vi "get#SamplesPerChannel.vi"(8 "error in (no error)":errorcluster, 10 "NIDAQmx data format":digitalwaveform[](array[waveform]), 11 "niDAQmxDO in":refnum<class "niDAQmxDO.lvclass">) -> (0 "error out":errorcluster, 1 "samplesPerChannel":i32, 2 "NIDAQmx data format out":digitalwaveform[](array[waveform]), 3 "niDAQmxDO out":refnum<class "niDAQmxDO.lvclass">)   [LabVIEW 2009, in "Hardware.lvlib" / "Channels.lvlib" / "niDAQmxDO.lvclass"]
uses:
  niDAQmxDO.lvclass
  <vilib>/Waveform/DWDTOps.llb/DWDT Digital to Boolean Array.vi
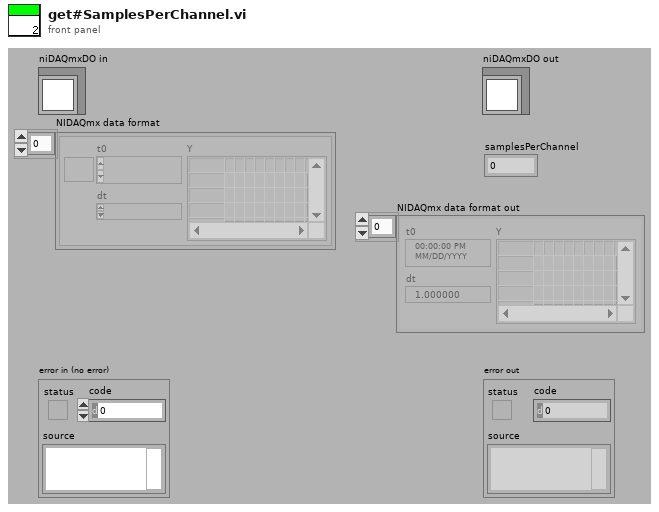
[diagram p1: front panel]
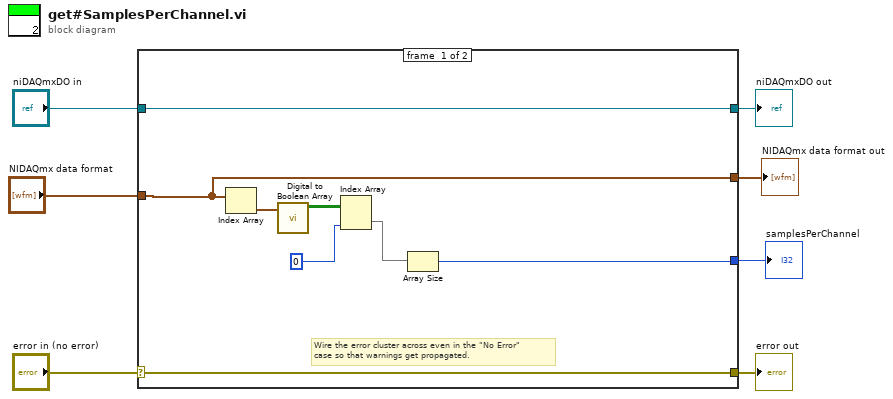
[diagram p0: block diagram]
diagram:
  n1 = case shown="No Error" "error in (no error)" {
    selector: "error in (no error)" -> [w14 w17]
    tunnel: [w14 w17] -> w6
    tunnel: [w15 w16] -> w4
    tunnel: "niDAQmxDO in" -> [w15 w16]
    tunnel: "NIDAQmx data format" -> [w8 _]
    tunnel: [w9 _] -> w2
    tunnel: [w8 _] -> w1
    frame #0 {
      # "Wire the error cluster across even in the \"No Error\"\ncase so that warnings get propagated."
      n2 = Index Array(array=w8) -> (element=w13:digitalwaveform)  [unwired: 1 in]
      n3 = call-poly <vilib>:"Digital to Boolean Array.vi"("digital waveform"=w13) -> ("boolean array"=w12:bool[][])  [unwired: 9 in, 1 out]
      n4 = Index Array(array=w12, index (col)=0) -> (element=w10:bool[])  [unwired: 1 in]
      n5 = Array Size(array=w10) -> (size(s)=w9:i32)
    }
    frame #1 {
    }
  }
  "error out" <- w6
  "niDAQmxDO out" <- w4
  "samplesPerChannel" <- w2
  "NIDAQmx data format out" <- w1
